vi "CH_LM VariantData2StreamingCluster.vi"(3 "error in (no error)":errorcluster, 5 "Streaming Data":variant[](array[variant])) -> (0 "error out":errorcluster, 2 "Streaming Data Cluster":T1 {"Flags" format="%.0b"; "Unit ID" format="%.0b"; "Quad Distance"."Y" format="%#.1f"; "Quad Distance"."X" format="%#.1f"; "Value" format="%#.7e"})   [LabVIEW 2017, in "CH_LM.lvlib"]
doc: "This VI converts the received USB streaming data record, Variant array, to Streaming Data Cluster."
uses:
  CH_LM.lvlib
  CH_LM/CH_LM Streaming Data.ctl
panel:
  in  "Steaming Data Cluster":T1 {"Flags" format="%.0b"; "Unit ID" format="%.0b"; "Quad Distance"."Y" format="%#.1f"; "Quad Distance"."X" format="%#.1f"; "Value" format="%#.7e"}
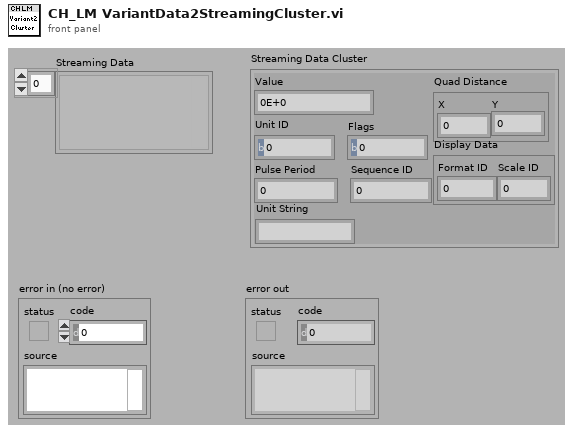
[diagram p1: front panel]
types:
  T1 = typedef "CH_LM.lvlib/CH_LM Streaming Data.ctl" = cluster{"Value":sgl, "Quad Distance":cluster{"X":sgl, "Y":sgl}, "Display Data":cluster{"Format ID":u8, "Scale ID":u8}, "Unit ID":u8, "Flags":u32, "Pulse Period":u32, "Sequence ID":u32, "Unit String":string}
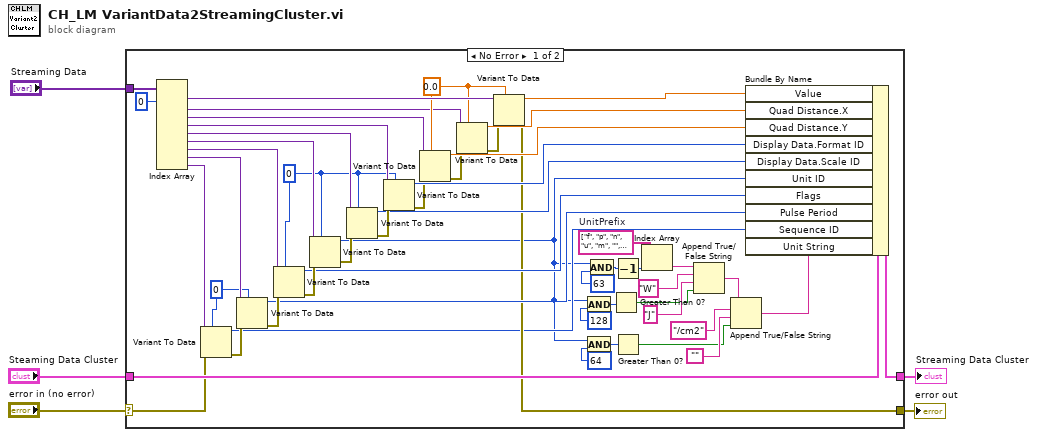
[diagram p0: block diagram]
diagram:
  n1 = case shown="No Error" "error in (no error)" {
    selector: "error in (no error)" -> [w26 w59]
    tunnel: [w25 w59] -> w3
    tunnel: "Steaming Data Cluster" -> [w51 w58]
    tunnel: [w50 w58] -> w1
    tunnel: "Streaming Data" -> [w57 _]
    frame No Error {
      w11 = string[] ["f", "p", "n", "u", "m", "", "k", "M", "G", "T", "P"]  # UnitPrefix
      w34 = u8 0
      w54 = sgl 0.0
      w28 = u32 0
      n2 = Index Array(array=w57, index #1=0 ("index")) -> (element #1=w55:variant, element #2=w53:variant, element #3=w52:variant, element #4=w46:variant, element #5=w44:variant, element #6=w37:variant, element #7=w35:variant, element #8=w30:variant, element #9=w29:variant)  [unwired: 8 in]
      n3 = Variant To Data(error in=w26, type=w28, Variant=w29) -> (data=w23:u32, error out=w31:errorcluster)
      n4 = Variant To Data(error in=w31, type=w28, Variant=w30) -> (data=w27:u32, error out=w32:errorcluster)
      n5 = Variant To Data(error in=w32, type=w34, Variant=w35) -> (data=w33:u8, error out=w36:errorcluster)
      n6 = Variant To Data(error in=w36, type=w34, Variant=w37) -> (data=w15:u8, error out=w38:errorcluster)
      n7 = Variant To Data(error in=w38, type=w34, Variant=w44) -> (data=w39:u8, error out=w40:errorcluster)
      n8 = Variant To Data(error in=w40, type=w34, Variant=w46) -> (data=w45:u8, error out=w41:errorcluster)
      n9 = Variant To Data(error in=w41, type=w54, Variant=w52) -> (data=w47:sgl, error out=w42:errorcluster)
      n10 = Variant To Data(error in=w42, type=w54, Variant=w53) -> (data=w48:sgl, error out=w43:errorcluster)
      n11 = Variant To Data(error in=w43, type=w54, Variant=w55) -> (data=w49:sgl, error out=w25:errorcluster)
      n12 = And(x=w15, y=u8 128 ("default value 1")) -> (x .and. y?=w24:u8)
      n13 = And(x=w15, y=u8 64 ("default value 1")) -> (x .and. y?=w18:u8)
      n14 = And(x=w15, y=u8 63 ("default value 1")) -> (x .and. y?=w13:u8)
      n15 = Greater Than 0?(x=w24) -> (x > 0?=w7:bool)
      n16 = Decrement(x=w13) -> (x-1=w12:u8)
      n17 = Greater Than 0?(x=w18) -> (x > 0?=w17:bool)
      n18 = Index Array(array=w11, index=w12) -> (element=w10:string)
      n19 = Append True/False String(1:w7, 2:"J" ("regular expression"), 3:"W" ("regular expression"), 4:w10) -> (0:w6:string)
      n20 = Append True/False String(1:w17, 2:"", 3:"/cm2" ("regular expression"), 4:w6) -> (0:w16:string)
      n21 = Bundle By Name(cluster=w51, "Value"=w49, "Quad Distance.X"=w48, "Quad Distance.Y"=w47, "Display Data.Format ID"=w45, "Display Data.Scale ID"=w39, "Unit ID"=w15, "Flags"=w33, "Pulse Period"=w27, "Sequence ID"=w23, "Unit String"=w16) -> (w50:T1)
    }
    frame Error {
    }
  }
  "error out" <- w3
  "Streaming Data Cluster" <- w1
